vi "KeyBindConceptTest.vi"() -> ()   [LabVIEW 2017]
panel:
  in  "Enums":dbl[](array[numeric])
  in  "Booleans":bool[](array[boolean])
  out "Output 5":bool=TRUE
  out "Output 4":bool=TRUE
  out "Output 3":bool=TRUE
  out "Output 2":bool=TRUE
  in  "Input 2":bool=TRUE
  out "Output":bool=TRUE
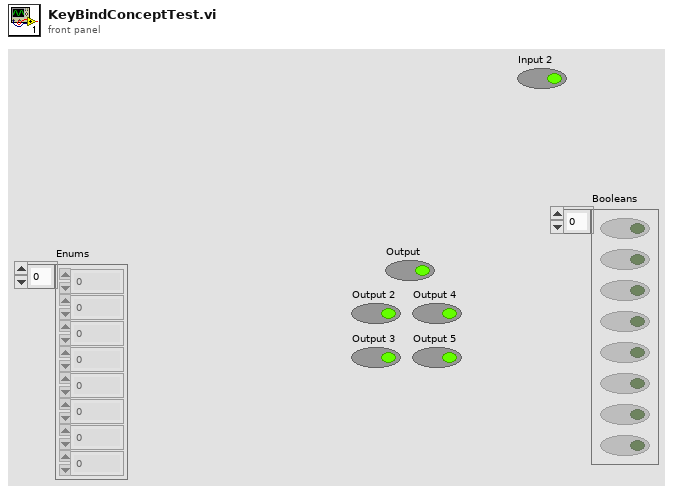
[diagram p1: front panel]
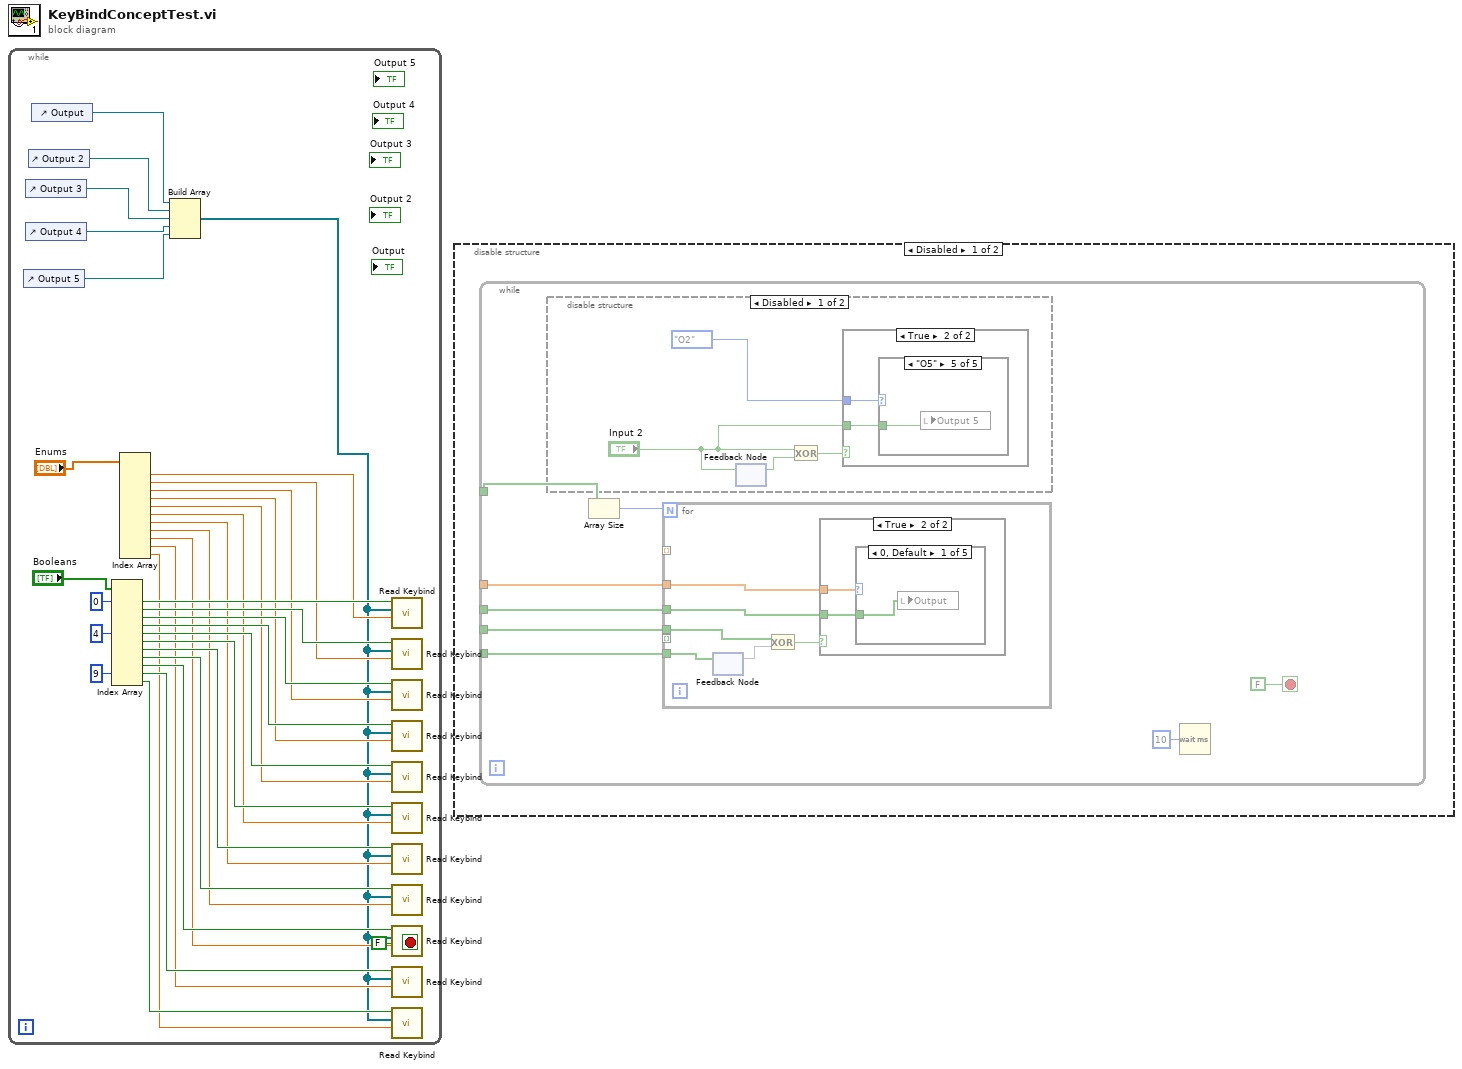
[diagram p0: block diagram]
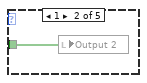
[diagram p3: hidden frame]
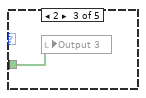
[diagram p4: hidden frame]
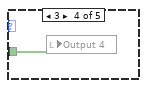
[diagram p5: hidden frame]
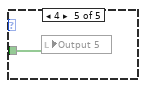
[diagram p6: hidden frame]
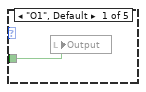
[diagram p8: hidden frame]
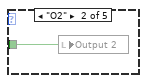
[diagram p9: hidden frame]
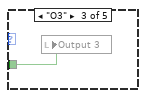
[diagram p10: hidden frame]
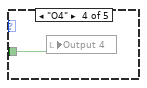
[diagram p11: hidden frame]
diagram:
  n1 = while {
    stop <- FALSE stop-if-true
    n2 = control-ref of="Output 5"() -> (w30:refnum<vi>)
    n3 = control-ref of="Output 3"() -> (w32:refnum<vi>)
    n4 = control-ref of="Output 4"() -> (w31:refnum<vi>)
    n5 = control-ref of="Output 2"() -> (w33:refnum<vi>)
    n6 = control-ref of="Output"() -> (w34:refnum<vi>)
    n7 = Index Array(array="Booleans", index #1=0 ("index"), index #5=4 ("index"), index #10=9 ("index")) -> (element #1=w25:bool, element #2=w24:bool, element #3=w23:bool, element #4=w22:bool, element #5=w20:bool, element #6=w19:bool, element #7=w18:bool, element #8=w17:bool, element #9=w16:bool, element #10=w15:bool, element #11=w14:bool)  [unwired: 8 in]
    n8 = Index Array(array="Enums") -> (element #1=w21:dbl, element #2=w13:dbl, element #3=w12:dbl, element #4=w11:dbl, element #5=w10:dbl, element #6=w9:dbl, element #7=w8:dbl, element #8=w7:dbl, element #9=w6:dbl, element #10=w5:dbl, element #11=w4:dbl)  [unwired: 11 in]
    n9 = Build Array(w34, w33, w32, w31, w30) -> (w3:refnum<vi>[])
    n10 = call "Read Keybind.vi"("Numeric"=w21, "appended array"=w3, "Boolean"=w25) -> ()  [unwired: 9 in]
    n11 = call "Read Keybind.vi"("Numeric"=w13, "appended array"=w3, "Boolean"=w24) -> ()  [unwired: 9 in]
    n12 = call "Read Keybind.vi"("Numeric"=w12, "appended array"=w3, "Boolean"=w23) -> ()  [unwired: 9 in]
    n13 = call "Read Keybind.vi"("Numeric"=w11, "appended array"=w3, "Boolean"=w22) -> ()  [unwired: 9 in]
    n14 = call "Read Keybind.vi"("Numeric"=w10, "appended array"=w3, "Boolean"=w20) -> ()  [unwired: 9 in]
    n15 = call "Read Keybind.vi"("Numeric"=w9, "appended array"=w3, "Boolean"=w19) -> ()  [unwired: 9 in]
    n16 = call "Read Keybind.vi"("Numeric"=w8, "appended array"=w3, "Boolean"=w18) -> ()  [unwired: 9 in]
    n17 = call "Read Keybind.vi"("Numeric"=w7, "appended array"=w3, "Boolean"=w17) -> ()  [unwired: 9 in]
    n18 = call "Read Keybind.vi"("Numeric"=w6, "appended array"=w3, "Boolean"=w16) -> ()  [unwired: 9 in]
    n19 = call "Read Keybind.vi"("Numeric"=w5, "appended array"=w3, "Boolean"=w15) -> ()  [unwired: 9 in]
    n20 = call "Read Keybind.vi"("Numeric"=w4, "appended array"=w3, "Boolean"=w14) -> ()  [unwired: 9 in]
  }
  n21 = disable-structure shown="Disabled" {
    frame Disabled {
      n22 = while {
        tunnel: _ -> [w39]
        tunnel: _ -> [w38]
        tunnel: _ -> [w37]
        tunnel: _ -> [w36]
        tunnel: _ -> [w35]
        stop <- FALSE stop-if-true
        n23 = disable-structure shown="Disabled" {
          frame Disabled {
            n24 = feedback #1() -> (w61:bool)  [unwired: 1 in]
            n25 = feedback-in #1("Input 2") -> ()
            n26 = Exclusive Or(1:w61, 2:"Input 2") -> (0:w60:bool)
            n27 = case shown="True" w60 {
              tunnel: "Input 2" -> [_ w63]
              tunnel: enum16{"O1", "O2", "O3", "O4", "O5"}."O2" -> [_ w62]
              frame False {
              }
              frame True {
                n28 = case shown="\"O5\"" w62 {
                  tunnel: w63 -> [w64 w65 w66 w67 w68]
                  frame "O1", Default {
                    n29 = local write "Output"(w64) -> ()
                  }
                  frame "O2" {
                    n30 = local write "Output 2"(w65) -> ()
                  }
                  frame "O3" {
                    n31 = local write "Output 3"(w66) -> ()
                  }
                  frame "O4" {
                    n32 = local write "Output 4"(w67) -> ()
                  }
                  frame "O5" {
                    n33 = local write "Output 5"(w68) -> ()
                  }
                }
              }
            }
          }
          frame Enabled {
          }
        }
        n34 = Array Size(array=w38) -> (size(s)=w41:i32)
        n35 = for {
          N: w41 -> [_]
          tunnel: _ -> [w48] mode=indexing
          tunnel: _ -> [w47] mode=indexing
          tunnel: w39 -> [w46]
          tunnel: w37 -> [w45]
          tunnel: w36 -> [w44]
          tunnel: w35 -> [w43]
          n36 = feedback #2() -> (w50)  [unwired: 1 in]
          n37 = feedback-in #2(w45) -> ()
          n38 = Exclusive Or(1:w50, 2:w43) -> (0:w49:bool)
          n39 = case shown="True" w49 {
            tunnel: w44 -> [_ w52]
            tunnel: w46 -> [_ w51]
            frame False {
            }
            frame True {
              n40 = case shown="0, Default" w51 {
                tunnel: w52 -> [w53 w54 w55 w56 w57]
                frame 0, Default {
                  n41 = local write "Output"(w53) -> ()
                }
                frame 1 {
                  n42 = local write "Output 2"(w54) -> ()
                }
                frame 2 {
                  n43 = local write "Output 3"(w55) -> ()
                }
                frame 3 {
                  n44 = local write "Output 4"(w56) -> ()
                }
                frame 4 {
                  n45 = local write "Output 5"(w57) -> ()
                }
              }
            }
          }
        }
        n46 = Wait (ms)(milliseconds to wait=u32 10) -> ()  [unwired: 1 out]
      }
    }
    frame Enabled {
    }
  }
